vi "Get and Set FP Bounds.vi"(7 "Select":enum16{"WinBounds", "PanelBounds"}(ring)=enum."PanelBounds", 8 "错误输入（无错误）":errorcluster, 9 "Mode":enum16{"Read", "Write"}(ring), 10 "Bounds In":T1, 11 "VI Ref In":refnum<vi>) -> (0 "错误输出":errorcluster, 2 "Bounds Out":T1, 3 "VI Ref Out":refnum<vi>)   [LabVIEW 2012, in "VIRef.lvlib"]
uses:
  VIRef.lvlib
  <vilib>/Utility/miscctls.llb/LVRectTypeDef.ctl
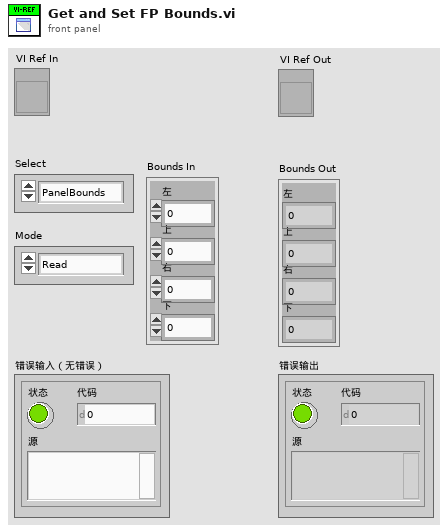
[diagram p1: front panel]
types:
  T1 = typedef "LVRectTypeDef.ctl" = cluster{"Left":i16, "Top":i16, "Right":i16, "Bottom":i16}
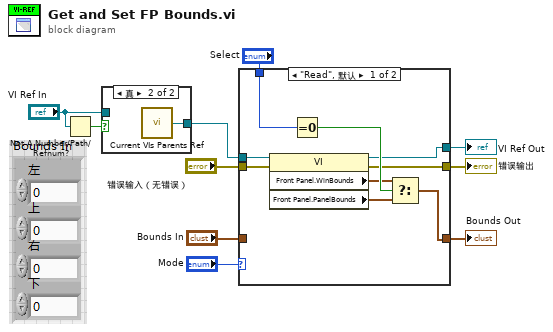
[diagram p0: block diagram]
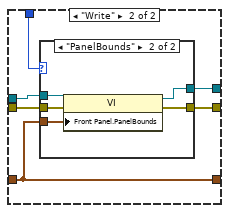
[diagram p2: hidden frame]
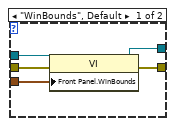
[diagram p3: hidden frame]
diagram:
  n1 = Not A Number/Path/Refnum?(number/path/refnum="VI Ref In") -> (NaN/Path/Refnum?=w10:bool)
  n2 = case shown="真" w10 {
    tunnel: [w11 w12] -> w3
    tunnel: "VI Ref In" -> [w11 _]
    frame False {
    }
    frame True {
      n3 = call "Current VIs Parents Ref.vi"() -> ("Calling VI's Reference"=w12:refnum<vi>)  [unwired: 2 in]
    }
  }
  n4 = case shown="\"Read\", 默认" "Mode" {
    tunnel: "Select" -> [w21 w27]
    tunnel: [w17 w22] -> w6
    tunnel: "错误输入（无错误）" -> [w16 w24]
    tunnel: [w15 w23] -> w4
    tunnel: w3 -> [w14 w26]
    tunnel: [w13 w25] -> w2
    tunnel: "Bounds In" -> [_ w22]
    frame "Read", Default {
      n5 = property class="VI"(reference=w14, error in=w16) -> (reference out=w13:refnum<vi>, error out=w15:errorcluster, "Front Panel.WinBounds"=w19:T1, "Front Panel.PanelBounds"=w18:T1)
      n6 = Equal To 0?(x=w21) -> (x = 0?=w20:bool)
      n7 = Select(t=w19, s=w20, f=w18) -> (s? t:f=w17:T1)
    }
    frame "Write" {
      n8 = case shown="\"PanelBounds\"" w27 {
        tunnel: w22 -> [w32 w37]
        tunnel: w26 -> [w31 w36]
        tunnel: [w30 w35] -> w25
        tunnel: w24 -> [w29 w34]
        tunnel: [w28 w33] -> w23
        frame "WinBounds", Default {
          n9 = property class="VI"(reference=w31, error in=w29, "Front Panel.WinBounds"=w32) -> (reference out=w30:refnum<vi>, error out=w28:errorcluster)
        }
        frame "PanelBounds" {
          n10 = property class="VI"(reference=w36, error in=w34, "Front Panel.PanelBounds"=w37) -> (reference out=w35:refnum<vi>, error out=w33:errorcluster)
        }
      }
    }
  }
  "VI Ref Out" <- w2
  "错误输出" <- w4
  "Bounds Out" <- w6
